vi "Compute Upper & Lower CI Plots.vi"(0 "Y Array":dbl[](array[numeric]), 1 "VI in":refnum<vi>, 3 "Additional LM Data":variant, 5 "X Array":dbl[](array[numeric]), 9 "Weight Array":dbl[](array[numeric]), 11 "error in (no error)":errorcluster, 12 "best fit parameters":dbl[](array[numeric]), 14 "confidence level (0.95)":dbl=0.95 format="%#_13g") -> (4 "CI Plots":T1[](array[typedef]), 15 "error out":errorcluster)   [LabVIEW 2021, in "Fits.lvlib"]
doc: "Computes the upper and lower confidence interval plots of a fit."
uses:
  Fits.lvlib
  Graphs/XY Graph/XY Graph Plot Data.ctl
  Graphs/XY Graph/XY Graph Add-Ons.lvlib
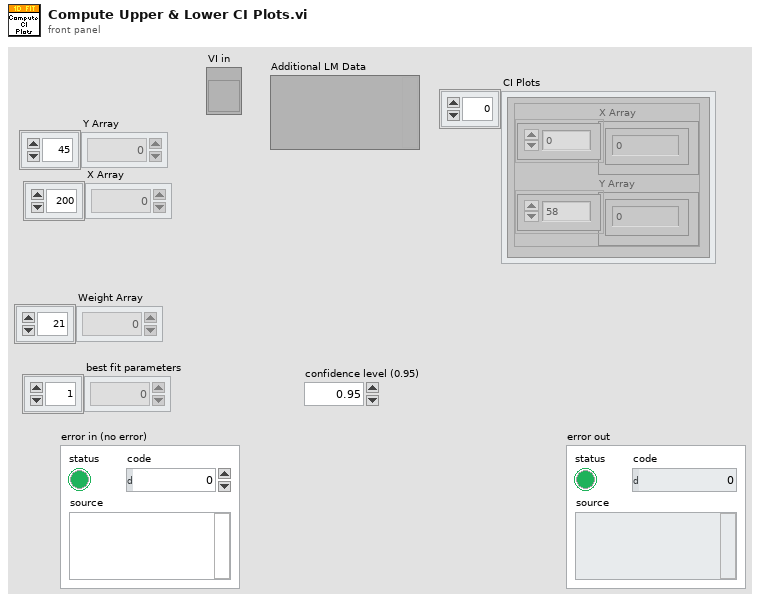
[diagram p1: front panel]
types:
  T1 = typedef "XY Graph Add-Ons.lvlib/XY Graph Plot Data.ctl" = cluster{"X Array":dbl[], "Y Array":dbl[]}
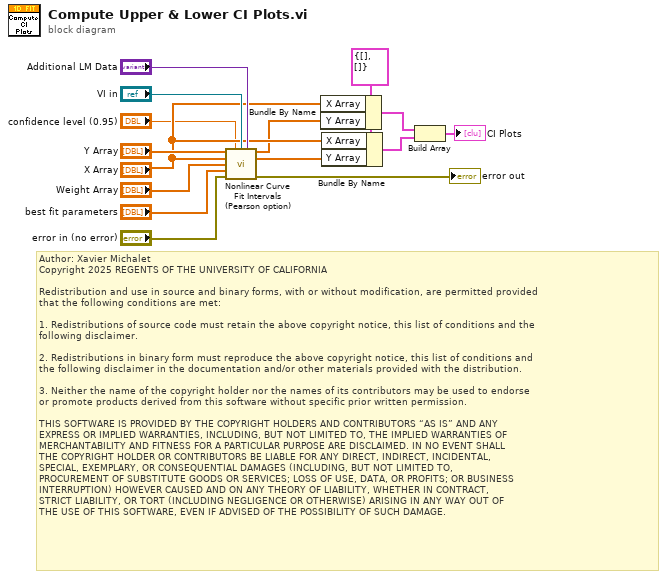
[diagram p0: block diagram]
diagram:
  w5 = T1 {"X Array"=[], "Y Array"=[]} ("Plot")
  # "Author: Xavier Michalet\nCopyright 2025 REGENTS OF THE UNIVERSITY OF CALIFORNIA\n\nRedistribution and use in source and binary forms, with or without modification, are permitted provided\nthat the following conditions are met:\n\n1. Redistributions of source code must retain the above copyright notice, this list of conditions and the\nfollowing disclaimer.\n\n2. Redistributions in binary form must reproduce the above copyright notice, this list of conditions and\nthe following disclaimer in the documentation and/or other materials provided with the distribution.\n\n3. Neither the name of the copyright holder nor the names of its contributors may be used to endorse \nor promote products derived from this software without specific prior written permission.\n\nTHIS SOFTWARE IS PROVIDED BY THE COPYRIGHT HOLDERS AND CONTRIBUTORS “AS IS” AND ANY \nEXPRESS OR IMPLIED WARRANTIES, INCLUDING, BUT NOT LIMITED TO, THE IMPLIED WARRANTIES OF\nMERCHANTABILITY AND FITNESS FOR A PARTICULAR PURPOSE ARE DISCLAIMED. IN NO EVENT SHALL\nTHE COPYRIGHT HOLDER OR CONTRIBUTORS BE LIABLE FOR ANY DIRECT, INDIRECT, INCIDENTAL, \nSPECIAL, EXEMPLARY, OR CONSEQUENTIAL DAMAGES (INCLUDING, BUT NOT LIMITED TO, \nPROCUREMENT OF SUBSTITUTE GOODS OR SERVICES; LOSS OF USE, DATA, OR PROFITS; OR BUSINESS\nINTERRUPTION) HOWEVER CAUSED AND ON ANY THEORY OF LIABILITY, WHETHER IN CONTRACT, \nSTRICT LIABILITY, OR TORT (INCLUDING NEGLIGENCE OR OTHERWISE) ARISING IN ANY WAY OUT OF\nTHE USE OF THIS SOFTWARE, EVEN IF ADVISED OF THE POSSIBILITY OF SUCH DAMAGE."
  n1 = call "Nonlinear Curve Fit Intervals (Pearson option).vi"("Y"="Y Array", "confidence level"="confidence level (0.95)", "f(x,a)"="VI in", "data"="Additional LM Data", "X"="X Array", "Weight"="Weight Array", "best fit parameters"="best fit parameters", "error in (no error)"="error in (no error)") -> ("Upper Bound"=w2:dbl[], "Lower Bound"=w1:dbl[], "error out"=→"error out":errorcluster)  [unwired: 4 in, 1 out]
  n2 = Bundle By Name(cluster=w5, "X Array"="X Array", "Y Array"=w2) -> (w9:T1)
  n3 = Bundle By Name(cluster=w5, "X Array"="X Array", "Y Array"=w1) -> (w8:T1)
  n4 = Build Array(w9, w8) -> (→"CI Plots":T1[])
